vi "InstrSlugFromIni.vi"(8 "error in (no error)":errorcluster, 11 "configuration file path":path=path "C:/BytelabsRepository/webapibytegs/RESTServerCfg.ini") -> (0 "error out":errorcluster, 3 "Array":string[](array[string]))   [LabVIEW 2019]
uses:
  <vilib>/Utility/config.llb/Read Key (String).vi
  <vilib>/Utility/config.llb/NI_LVConfig.lvlib
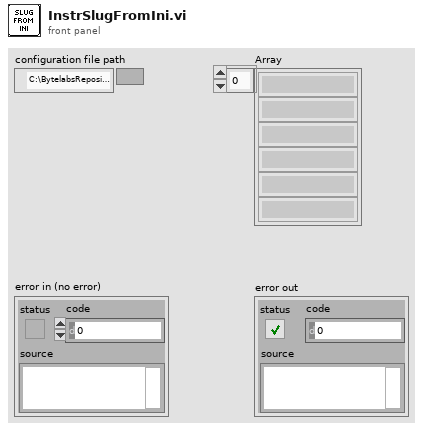
[diagram p1: front panel]
types:
  T1 = typedef "NI_LVConfig.lvlib/Config Data RefNum.ctl" = refnum<k1>
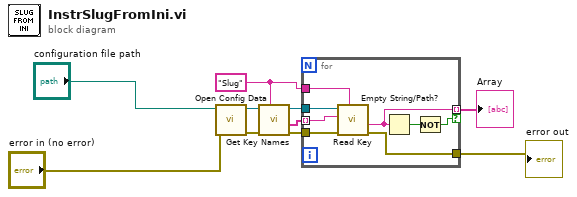
[diagram p0: block diagram]
diagram:
  w6 = "Slug" ("section")
  n1 = call <vilib>:"Open Config Data.vi"("error in (no error)"="error in (no error)", "configuration file path"="configuration file path") -> ("error out"=w5:errorcluster, "refnum"=w9:T1)  [unwired: 7 in, 1 out]
  n2 = call <vilib>:"Get Key Names.vi"("section"=w6, "error in (no error)"=w5, "refnum"=w9) -> ("error out"=w4:errorcluster, "key names"=w3:string[], "refnum out"=w7:T1)  [unwired: 5 in, 1 out]
  n3 = for {
    tunnel: w7 -> [w18]
    tunnel: w4 -> [w17]
    tunnel: [w14] -> w8 mode=indexing if=w12
    tunnel: w6 -> [w16]
    tunnel: w3 -> [w15] mode=indexing
    tunnel: [w11] -> w1
    n4 = call-poly <vilib>:"Read Key.vi"("section"=w16, "error in (no error)"=w17, "key"=w15, "refnum"=w18) -> ("error out"=w11:errorcluster, "value"=w14:string)  [unwired: 4 in, 2 out]
    n5 = Empty String/Path?(string/path=w14) -> (empty?=w13:bool)
    n6 = Not(x=w13) -> (.not. x?=w12:bool)
  }
  "Array" <- w8
  "error out" <- w1
